vi "sub_step_FIXED.vi"(2 "Current Position":i32, 3 "millisecond multiple":u32=10, 4 "Desired Position":i32) -> (1 "Position Out":i32)   [LabVIEW 2014]
panel:
  out "Current Position {RUN}":i32
  in  "stop":bool
  # "In Stepper\nMotor\nSteps"
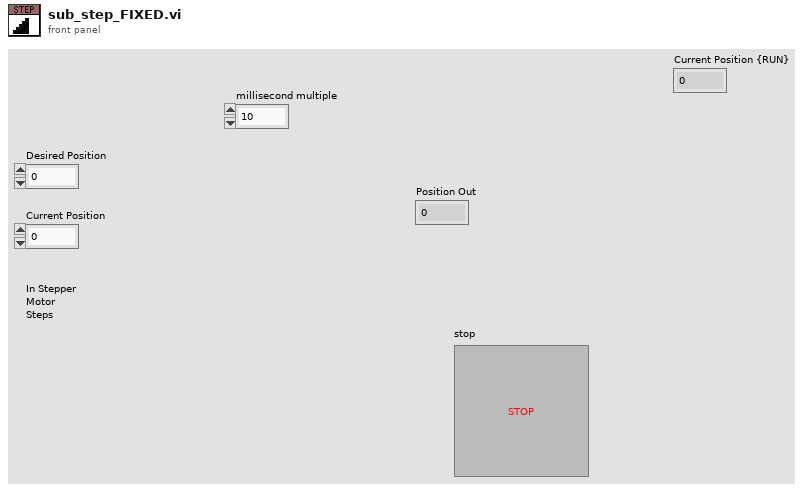
[diagram p1: front panel]
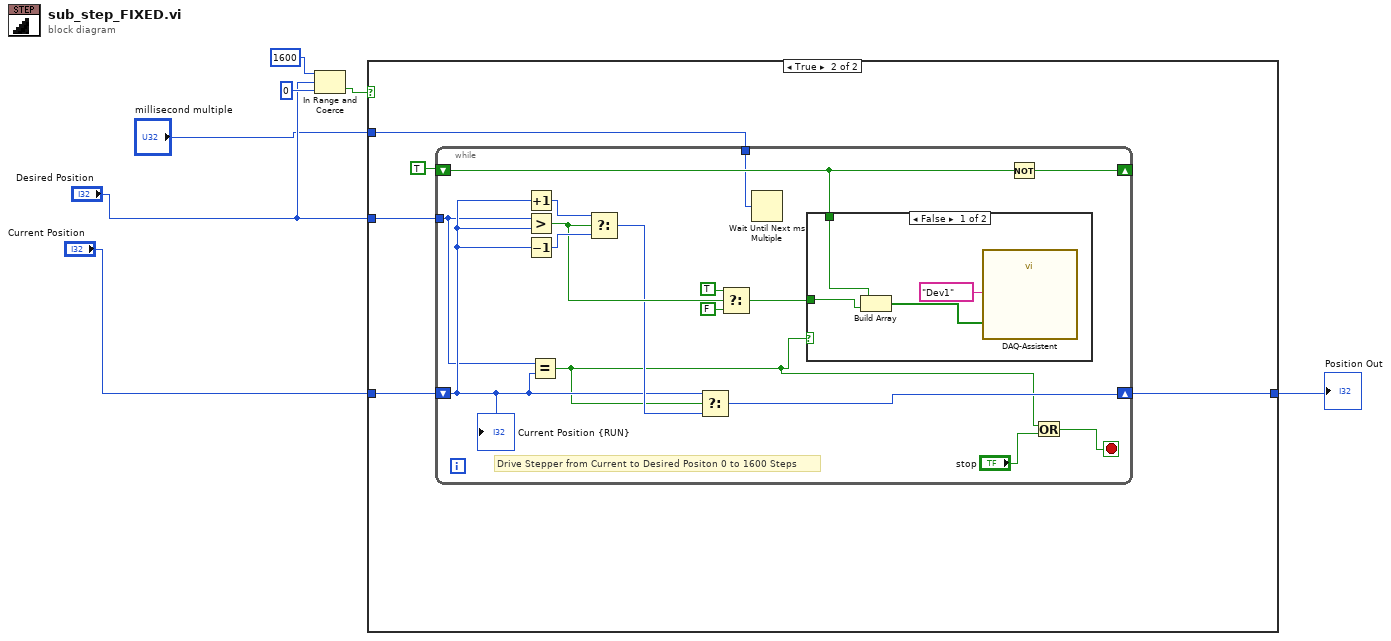
[diagram p0: block diagram]
diagram:
  n1 = In Range and Coerce(upper limit=1600, x="Desired Position", lower limit=0) -> (In Range?=w6:bool)  [unwired: 1 out]
  n2 = case shown="True" w6 {
    tunnel: [w8 w13] -> w7
    tunnel: "Current Position" -> [w8 w11]
    tunnel: "Desired Position" -> [_ w10]
    tunnel: "millisecond multiple" -> [_ w9]
    frame False {
    }
    frame True {
      n3 = while {
        shift-right: [w21] -> w13
        shift-left: w11 -> [w22]
        shift-right: [w20] -> _
        shift-left: TRUE -> [w19]
        tunnel: w10 -> [w18]
        tunnel: w9 -> [w14]
        stop <- w15 stop-if-true
        # "Drive Stepper from Current to Desired Positon 0 to 1600 Steps"
        n4 = Increment(x=w22) -> (x+1=w26:i32)
        n5 = Greater?(x=w18, y=w22) -> (0:w24:bool)
        n6 = Decrement(x=w22) -> (x-1=w25:i32)
        n7 = Equal?(x=w18, y=w22) -> (x = y?=w16:bool)
        n8 = Select(t=w26, s=w24, f=w25) -> (s? t:f=w23:i32)
        n9 = Select(t=w22, s=w16, f=w23) -> (s? t:f=w21:i32)
        n10 = Select(t=TRUE, s=w24, f=FALSE) -> (s? t:f=w29:bool)
        n11 = Wait Until Next ms Multiple(millisecond multiple=w14) -> ()  [unwired: 1 out]
        n12 = case shown="False" w16 {
          tunnel: w29 -> [w33 _]
          tunnel: w19 -> [w32 _]
          frame False {
            n13 = Build Array(w32, w33) -> (w31:bool[])
            n14 = call "DAQ-Assistent"("data"=w31, "device name"=tag "Dev1") -> ()  [unwired: 16 in, 2 out]
          }
          frame True {
          }
        }
        n15 = Not(x=w19) -> (.not. x?=w20:bool)
        n16 = Or(x=w16, y="stop") -> (x .or. y?=w15:bool)
        "Current Position {RUN}" <- w22
      }
    }
  }
  "Position Out" <- w7
